vi "Q Learning (Demo).vi"() -> ()   [LabVIEW 2013]
panel:
  out "Q":dbl[][](array[numeric])
  in  "stop":bool
  # "Next Room"
  # "Current Room"
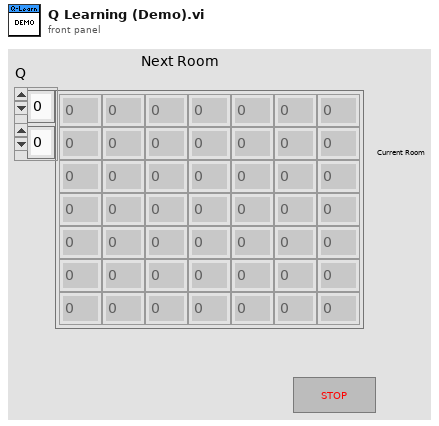
[diagram p1: front panel]
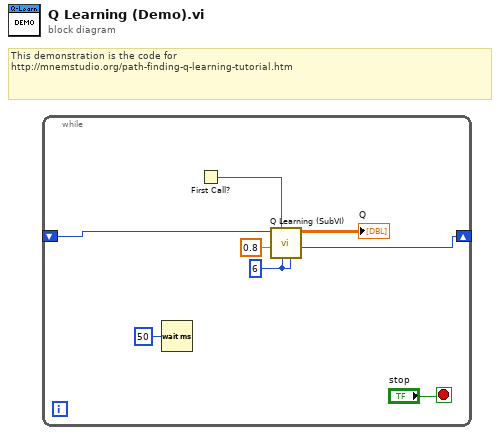
[diagram p0: block diagram]
diagram:
  # "This demonstration is the code for \nhttp://mnemstudio.org/path-finding-q-learning-tutorial.htm"
  n1 = while {
    shift-right: [w3] -> _
    shift-left: _ -> [w6]
    stop <- "stop" stop-if-true
    w7 = 6 ("# state")
    n2 = Wait (ms)(milliseconds to wait=u32 50) -> ()  [unwired: 1 out]
    n3 = First Call?() -> (First Call?: T/F=w2:bool)
    n4 = call "Q Learning (SubVI).vi"("# action"=w7, "# state"=w7, "Reset"=w2, "Gamma"=0.8, "State"=w6) -> ("Next Action"=w3:i32, "Q"=→"Q":dbl[][])  [unwired: 5 in]
  }
